vi "FOCUS_V42_H37.vi"(9 "X-pixels":sgl=256.0, 11 "Run":bool) -> (0 "Retrace pixels":sgl, 10 "Pixel Clock (Hz)":sgl)   [LabVIEW 2010] (continued)
                  n1368 = property on="index (row)1" class="Slide (strict)"("Scale.Range:Minimum"=w941, "Scale.Range:Maximum"=w942) -> ()  [unwired: 2 in, 2 out]
                  n1369 = Add(x=w957, y=w958) -> (x+y=w956:dbl)
                  n1370 = property on="Histogram2" class="XYGraph (strict)"("X Scale.Range:Minimum"=w957, "X Scale.Range:Maximum"=w956) -> ()  [unwired: 2 in, 2 out]
                  n1371 = property on="Histogram1" class="XYGraph (strict)"("X Scale.Range:Minimum"=w957, "X Scale.Range:Maximum"=w956) -> ()  [unwired: 2 in, 2 out]
                  n1372 = Initialize Array(u32 0 ("element"), w892) -> (w950:u32[])
                  n1373 = Array Subset(array=w888, index (row)=w903, length (row)=w902) -> (w948:u8[][])  [unwired: 2 in]
                  n1374 = Initialize Array(u32 0 ("element"), w892) -> (w954:u32[])
                  n1375 = Array Subset(array=w887, index (row)=w901, length (row)=w900) -> (w952:u8[][])  [unwired: 2 in]
                  n1376 = property on="index (row)2" class="Slide (strict)"("Scale.Range:Minimum"=w941, "Scale.Range:Maximum"=w940) -> ()  [unwired: 2 in, 2 out]
                  n1377 = local read "Background1"() -> (w914:bool)
                  n1378 = for {
                    tunnel: w948 -> [w1025] mode=indexing
                    shift-right: [w1024] -> w949
                    shift-left: w950 -> [w1026]
                    n1379 = Add(x=w1026, y=w1025) -> (x+y=w1024:u32[])
                  }
                  n1380 = local read "Index1"() -> (w928:dbl)
                  n1381 = local read "Length1"() -> (w929:dbl)
                  n1382 = for {
                    tunnel: w952 -> [w1022] mode=indexing
                    shift-right: [w1021] -> w953
                    shift-left: w954 -> [w1023]
                    n1383 = Add(x=w1023, y=w1022) -> (x+y=w1021:u32[])
                  }
                  n1384 = local read "X-pixels"() -> (w890:sgl)
                  n1385 = local read "Pixel Clock (Hz)"() -> (w946:sgl)
                  n1386 = Divide(x=w949, y=w902) -> (x/y=w891:dbl[])
                  n1387 = Array Subset(array=w891, index=w928, length=w929) -> (w925:dbl[])
                  n1388 = Divide(x=w953, y=w900) -> (x/y=w931:dbl[])
                  n1389 = Array Subset(array=w888, index (row)=w957, length (row)=w958, index (col)=w904, length (col)=w889) -> (w960:u8[][])
                  n1390 = Array Subset(array=w887, index (row)=w957, length (row)=w958, index (col)=w904, length (col)=w889) -> (w959:u8[][])
                  n1391 = case shown="True" w914 {
                    tunnel: w891 -> [_ w968]
                    frame False {
                    }
                    frame True {
                      n1392 = Array Size(array=w968) -> (size(s)=w969:i32)
                      n1393 = Add Array Elements(numeric array=w968) -> (sum=w970:dbl)
                      n1394 = Divide(x=w970, y=w969) -> (x/y=w967:dbl)
                      n1395 = local write "Background1 2"(w967) -> ()
                    }
                  }
                  n1396 = Array Size(array=w925) -> (size(s)=w927:i32)
                  n1397 = Add Array Elements(numeric array=w925) -> (sum=w926:dbl)
                  n1398 = Divide(x=w890, y=w946) -> (x/y=w945:sgl)
                  n1399 = local write "Image 1"(w960) -> ()
                  n1400 = Divide(x=w926, y=w927) -> (x/y=w913:dbl)
                  n1401 = local write "Image 2"(w959) -> ()
                  n1402 = local write "F01 2"(w913) -> ()
                  n1403 = Multiply(x=1000.0, y=w945) -> (x*y=w895:dbl)
                  n1404 = Multiply(x=w892, y=w895) -> (x*y=w937:dbl)
                  n1405 = case shown="True" w915 {
                    tunnel: w937 -> [_ w1020]
                    frame False {
                    }
                    frame True {
                      n1406 = property on="Profile1" class="XYGraph (strict)"("X Scale.Range:Minimum"=0.0, "X Scale.Range:Maximum"=w1020, "Y Scale.Range:Minimum"=0.0, "Y Scale.Range:Maximum"=255.0) -> ()  [unwired: 2 in, 2 out]
                    }
                  }
                  n1407 = case shown="True" w916 {
                    tunnel: w937 -> [_ w997]
                    frame False {
                    }
                    frame True {
                      n1408 = property on="Profile2" class="XYGraph (strict)"("X Scale.Range:Minimum"=0.0, "X Scale.Range:Maximum"=w997, "Y Scale.Range:Minimum"=0.0, "Y Scale.Range:Maximum"=255.0) -> ()  [unwired: 2 in, 2 out]
                    }
                  }
                  n1409 = local read "F0 1"() -> (w908:bool)
                  n1410 = Multiply(x=w895, y=w943) -> (x*y=w897:dbl[])
                  n1411 = Multiply(x=w895, y=w943) -> (x*y=w955:dbl[])
                  n1412 = local read "F0 2"() -> (w909:bool)
                  n1413 = local read "Background2"() -> (w911:bool)
                  n1414 = case shown="True" w909 {
                    tunnel: w931 -> [w1001 w1015]
                    tunnel: [w1001 w1007] -> w939
                    tunnel: w905 -> [w1000 _]
                    tunnel: [w998 i8 -1 ("Active Cursor")] -> w938
                    frame False {
                      n1415 = Less Than 0?(x=w1000) -> (x < 0?=w999:bool)
                      n1416 = case shown="False" w999 {
                        selector: w999 -> [w1003 w1005]
                        tunnel: [i8 1 ("Active Cursor") i8 1 ("Active Cursor")] -> w998
                        frame False {
                          n1417 = local write "Reset2"(w1003) -> ()
                        }
                        frame True {
                          n1418 = local write "Reset2"(w1005) -> ()
                        }
                      }
                    }
                    frame True {
                      n1419 = local read "Background2 2"() -> (w1013:sgl)
                      n1420 = local read "F02 2"() -> (w1010:sgl)
                      n1421 = Subtract(x=w1015, y=w1010) -> (x-y=w1014:dbl[])
                      n1422 = Subtract(x=w1010, y=w1013) -> (x-y=w1016:sgl)
                      n1423 = Divide(x=w1014, y=w1016) -> (x/y=w1008:dbl[])
                      n1424 = property on="Profile2" class="XYGraph (strict)"("Y Scale.Range:Minimum"=-100.0, "Y Scale.Range:Maximum"=100.0) -> ()  [unwired: 2 in, 2 out]
                      n1425 = Multiply(x=w1008, y=100.0 ("Y Scale.Range:Maximum")) -> (x*y=w1007:dbl[])
                    }
                  }
                  n1426 = case shown="True" w908 {
                    tunnel: w891 -> [w974 w988]
                    tunnel: [w974 w980] -> w896
                    tunnel: w906 -> [w973 _]
                    tunnel: [w971 i8 -1 ("Active Cursor")] -> w930
                    frame False {
                      n1427 = Less Than 0?(x=w973) -> (x < 0?=w972:bool)
                      n1428 = case shown="True" w972 {
                        selector: w972 -> [w976 w978]
                        tunnel: [i8 1 ("Active Cursor") i8 1 ("Active Cursor")] -> w971
                        frame False {
                          n1429 = local write "Reset1"(w976) -> ()
                        }
                        frame True {
                          n1430 = local write "Reset1"(w978) -> ()
                        }
                      }
                    }
                    frame True {
                      n1431 = local read "Background1 2"() -> (w986:sgl)
                      n1432 = local read "F01 2"() -> (w983:sgl)
                      n1433 = Subtract(x=w988, y=w983) -> (x-y=w987:dbl[])
                      n1434 = Subtract(x=w983, y=w986) -> (x-y=w989:sgl)
                      n1435 = Divide(x=w987, y=w989) -> (x/y=w981:dbl[])
                      n1436 = property on="Profile1" class="XYGraph (strict)"("Y Scale.Range:Minimum"=-100.0, "Y Scale.Range:Maximum"=100.0) -> ()  [unwired: 2 in, 2 out]
                      n1437 = Multiply(x=w981, y=100.0 ("Y Scale.Range:Maximum")) -> (x*y=w980:dbl[])
                    }
                  }
                  n1438 = property on="Profile2" class="XYGraph (strict)"() -> ("X Scale.Range:Minimum"=w920:dbl, "X Scale.Range:Maximum"=w919:dbl)  [unwired: 2 in, 2 out]
                  n1439 = local read "Index2"() -> (w933:dbl)
                  n1440 = local read "Length2"() -> (w932:dbl)
                  n1441 = property on="Profile1" class="XYGraph (strict)"() -> ("X Scale.Range:Minimum"=w921:dbl, "X Scale.Range:Maximum"=w922:dbl)  [unwired: 2 in, 2 out]
                  n1442 = case shown="True" w911 {
                    tunnel: w931 -> [_ w991]
                    frame False {
                    }
                    frame True {
                      n1443 = Array Size(array=w991) -> (size(s)=w992:i32)
                      n1444 = Add Array Elements(numeric array=w991) -> (sum=w993:dbl)
                      n1445 = Divide(x=w993, y=w992) -> (x/y=w990:dbl)
                      n1446 = local write "Background2 2"(w990) -> ()
                    }
                  }
                  n1447 = Array Subset(array=w931, index=w933, length=w932) -> (w936:dbl[])
                  n1448 = local read "F02"() -> (w907:bool)
                  n1449 = local read "F01"() -> (w912:bool)
                  n1450 = Divide(x=w920, y=w895) -> (x/y=w918:dbl)
                  n1451 = Divide(x=w919, y=w895) -> (x/y=w917:dbl)
                  n1452 = Divide(x=w921, y=w895) -> (x/y=w923:dbl)
                  n1453 = Divide(x=w922, y=w895) -> (x/y=w924:dbl)
                  n1454 = Array Size(array=w936) -> (size(s)=w934:i32)
                  n1455 = Add Array Elements(numeric array=w936) -> (sum=w935:dbl)
                  n1456 = case shown="True" w907 {
                    tunnel: w918 -> [_ w962]
                    tunnel: w917 -> [_ w963]
                    frame False {
                    }
                    frame True {
                      n1457 = local write "Index2"(w962) -> ()
                      n1458 = Subtract(x=w963, y=w962) -> (x-y=w961:dbl)
                      n1459 = local write "Length2"(w961) -> ()
                    }
                  }
                  n1460 = case shown="True" w912 {
                    tunnel: w923 -> [_ w965]
                    tunnel: w924 -> [_ w966]
                    frame False {
                    }
                    frame True {
                      n1461 = Subtract(x=w966, y=w965) -> (x-y=w964:dbl)
                      n1462 = local write "Index1"(w965) -> ()
                      n1463 = local write "Length1"(w964) -> ()
                    }
                  }
                  n1464 = Divide(x=w935, y=w934) -> (x/y=w910:dbl)
                  n1465 = local write "F02 2"(w910) -> ()
                  n1466 = Bundle(w955, w939) -> (w899:cluster{dbl[], dbl[]})  [unwired: 1 in]
                  n1467 = local write "Profile2"(w899) -> ()
                  n1468 = Bundle(w897, w896) -> (w898:cluster{dbl[], dbl[]})  [unwired: 1 in]
                  n1469 = local write "Profile1"(w898) -> ()
                }
                frame True {
                  n1470 = local read "Y-Scale"() -> (w1029:bool)
                  n1471 = case shown="False" w1029 {
                    tunnel: w1028 -> [w1031 _]
                    tunnel: w1027 -> [w1030 _]
                    frame False {
                      n1472 = local read "Y-lines"() -> (w1033:sgl)
                      n1473 = local read "Number of frames"() -> (w1034:sgl)
                      n1474 = local read "X-pixels"() -> (w1036:sgl)
                      n1475 = Multiply(x=w1034, y=w1033) -> (x*y=w1032:sgl)
                      n1476 = Subtract(x=w1032, y=w1036) -> (x-y=w1035:sgl)
                      n1477 = while {
                        shift-right: [w1045] -> _
                        shift-left: i16 0 ("y") -> [w1046]
                        tunnel: w1035 -> [w1044]
                        tunnel: w1031 -> [w1039]
                        tunnel: w1030 -> [w1038]
                        stop <- w1042 stop-if-true
                        n1478 = call "ResetToZeroFOCUS.vi"("UpperLimit"=w1044, "Running Index"=w1046) -> ("New Index"=w1040:i32)
                        n1479 = local read "Play Movie"() -> (w1043:bool)
                        n1480 = local write "ImageSlide"(w1040) -> ()
                        n1481 = local read "X-pixels"() -> (w1049:sgl)
                        n1482 = Not(x=w1043) -> (.not. x?=w1042:bool)
                        n1483 = Increment(x=w1040) -> (x+1=w1045:i32)
                        n1484 = local read "Velocity"() -> (w1041:dbl)
                        n1485 = Array Subset(array=w1039, index (col)=w1040, length (col)=w1049) -> (w1048:u8[][])  [unwired: 2 in]
                        n1486 = Array Subset(array=w1038, index (col)=w1040, length (col)=w1049) -> (w1047:u8[][])  [unwired: 2 in]
                        n1487 = Wait Until Next ms Multiple(millisecond multiple=w1041) -> ()  [unwired: 1 out]
                        n1488 = local write "Image 1"(w1048) -> ()
                        n1489 = local write "Image 2"(w1047) -> ()
                      }
                    }
                    frame True {
                    }
                  }
                }
              }
            }
            frame 3 {
              n1490 = case shown="False" w1056 {
                tunnel: w1055 -> [_ _]
                tunnel: w1061 -> [w1120 _]
                tunnel: [w1114 _] -> w1058
                tunnel: [w1106 _] -> w1057
                tunnel: w1060 -> [w1075 _]
                tunnel: w1059 -> [w1074 _]
                tunnel: w1054 -> [w1066 _]
                tunnel: w1053 -> [w1065 w1206]
                tunnel: w1052 -> [w1064 w1205]
                tunnel: w1051 -> [w1063 _]
                tunnel: w1050 -> [w1062 _]
                frame False {
                  w1067 = 0 ("index")
                  w1135 = 0.0
                  w1118 = 0.0 ("Scale.Range:Minimum")
                  n1491 = local read "Reset1"() -> (w1090:bool)
                  n1492 = local read "Reset2"() -> (w1091:bool)
                  n1493 = local read "Y-lines FreeLine"() -> (w1116:sgl)
                  n1494 = local read "X-pixels FreeLine"() -> (w1136:sgl)
                  n1495 = Add(x=w1135, y=w1136) -> (x+y=w1134:dbl)
                  n1496 = property on="Histogram2" class="XYGraph (strict)"("X Scale.Range:Minimum"=w1135, "X Scale.Range:Maximum"=w1134) -> ()  [unwired: 2 in, 2 out]
                  n1497 = property on="Histogram1" class="XYGraph (strict)"("X Scale.Range:Minimum"=w1135, "X Scale.Range:Maximum"=w1134) -> ()  [unwired: 2 in, 2 out]
                  n1498 = Initialize Array(u32 0 ("element"), w1116) -> (w1128:u32[])
                  n1499 = Array Subset(array=w1065, index (row)="index (row)1", length (row)="Average1") -> (w1126:u8[][])  [unwired: 2 in]
                  n1500 = Initialize Array(u32 0 ("element"), w1116) -> (w1132:u32[])
                  n1501 = Array Subset(array=w1064, index (row)="index (row)2", length (row)="Average2") -> (w1130:u8[][])  [unwired: 2 in]
                  n1502 = local read "Background1"() -> (w1089:bool)
                  n1503 = for {
                    tunnel: w1126 -> [w1203] mode=indexing
                    shift-right: [w1202] -> w1127
                    shift-left: w1128 -> [w1204]
                    n1504 = Add(x=w1204, y=w1203) -> (x+y=w1202:u32[])
                  }
                  n1505 = local read "Index1"() -> (w1104:dbl)
                  n1506 = local read "Length1"() -> (w1105:dbl)
                  n1507 = for {
                    tunnel: w1130 -> [w1200] mode=indexing
                    shift-right: [w1199] -> w1131
                    shift-left: w1132 -> [w1201]
                    n1508 = Add(x=w1201, y=w1200) -> (x+y=w1199:u32[])
                  }
                  n1509 = local read "X-pixels FreeLine"() -> (w1068:sgl)
                  n1510 = Subtract(x=w1068, y="Average2") -> (x-y=w1117:sgl)
                  n1511 = Subtract(x=w1068, y="Average1") -> (x-y=w1119:sgl)
                  n1512 = property on="index (row)1" class="Slide (strict)"("Scale.Range:Minimum"=w1118, "Scale.Range:Maximum"=w1119) -> ()  [unwired: 2 in, 2 out]
                  n1513 = property on="index (row)2" class="Slide (strict)"("Scale.Range:Minimum"=w1118, "Scale.Range:Maximum"=w1117) -> ()  [unwired: 2 in, 2 out]
                  n1514 = local read "Pixel Clock (Hz) FreeLine"() -> (w1124:sgl)
                  n1515 = Divide(x=w1127, y="Average1") -> (x/y=w1073:dbl[])
                  n1516 = Array Subset(array=w1073, index=w1104, length=w1105) -> (w1101:dbl[])
                  n1517 = Divide(x=w1131, y="Average2") -> (x/y=w1107:dbl[])
                  n1518 = Array Subset(array=w1065, index (row)=w1135, length (row)=w1136, index (col)=w1066, length (col)=w1068) -> (w1138:u8[][])
                  n1519 = Array Subset(array=w1064, index (row)=w1135, length (row)=w1136, index (col)=w1066, length (col)=w1068) -> (w1137:u8[][])
                  n1520 = case shown="True" w1089 {
                    tunnel: w1073 -> [_ w1146]
                    frame False {
                    }
                    frame True {
                      n1521 = Array Size(array=w1146) -> (size(s)=w1147:i32)
                      n1522 = Add Array Elements(numeric array=w1146) -> (sum=w1148:dbl)
                      n1523 = Divide(x=w1148, y=w1147) -> (x/y=w1145:dbl)
                      n1524 = local write "Background1 2"(w1145) -> ()
                    }
                  }
                  n1525 = Array Size(array=w1101) -> (size(s)=w1103:i32)
                  n1526 = Add Array Elements(numeric array=w1101) -> (sum=w1102:dbl)
                  n1527 = Divide(x=w1068, y=w1124) -> (x/y=w1123:sgl)
                  n1528 = local write "Image 3"(w1138) -> ()
                  n1529 = Divide(x=w1102, y=w1103) -> (x/y=w1088:dbl)
                  n1530 = local write "Image 4"(w1137) -> ()
                  n1531 = local write "F01 2"(w1088) -> ()
                  n1532 = Multiply(x=1000.0, y=w1123) -> (x*y=w1092:dbl)
                  n1533 = Multiply(x=w1116, y=w1092) -> (x*y=w1113:dbl)
                  n1534 = case shown="True" w1090 {
                    tunnel: w1113 -> [_ w1198]
                    frame False {
                    }
                    frame True {
                      n1535 = property on="Profile1" class="XYGraph (strict)"("X Scale.Range:Minimum"=0.0, "X Scale.Range:Maximum"=w1198, "Y Scale.Range:Minimum"=0.0, "Y Scale.Range:Maximum"=255.0) -> ()  [unwired: 2 in, 2 out]
                    }
                  }
                  n1536 = case shown="True" w1091 {
                    tunnel: w1113 -> [_ w1175]
                    frame False {
                    }
                    frame True {
                      n1537 = property on="Profile2" class="XYGraph (strict)"("X Scale.Range:Minimum"=0.0, "X Scale.Range:Maximum"=w1175, "Y Scale.Range:Minimum"=0.0, "Y Scale.Range:Maximum"=255.0) -> ()  [unwired: 2 in, 2 out]
                    }
                  }
                  n1538 = local read "Y-lines"() -> (w1069:sgl)
                  n1539 = local read "F0 1"() -> (w1083:bool)
                  n1540 = Multiply(x=w1092, y=w1120) -> (x*y=w1121:dbl[])
                  n1541 = Multiply(x=w1092, y=w1120) -> (x*y=w1133:dbl[])
                  n1542 = local read "F0 2"() -> (w1084:bool)
                  n1543 = local read "Background2"() -> (w1086:bool)
                  n1544 = case shown="True" w1084 {
                    tunnel: w1107 -> [w1179 w1193]
                    tunnel: [w1179 w1185] -> w1115
                    tunnel: w1074 -> [w1178 _]
                    tunnel: [w1176 i8 -1 ("Active Cursor")] -> w1114
                    frame False {
                      n1545 = Less Than 0?(x=w1178) -> (x < 0?=w1177:bool)
                      n1546 = case shown="True" w1177 {
                        selector: w1177 -> [w1181 w1183]
                        tunnel: [i8 1 ("Active Cursor") i8 1 ("Active Cursor")] -> w1176
                        frame False {
                          n1547 = local write "Reset2"(w1181) -> ()
                        }
                        frame True {
                          n1548 = local write "Reset2"(w1183) -> ()
                        }
                      }
                    }
                    frame True {
                      n1549 = local read "Background2 2"() -> (w1191:sgl)
                      n1550 = local read "F02 2"() -> (w1188:sgl)
                      n1551 = Subtract(x=w1193, y=w1188) -> (x-y=w1192:dbl[])
                      n1552 = Subtract(x=w1188, y=w1191) -> (x-y=w1194:sgl)
                      n1553 = Divide(x=w1192, y=w1194) -> (x/y=w1186:dbl[])
                      n1554 = property on="Profile2" class="XYGraph (strict)"("Y Scale.Range:Minimum"=-100.0, "Y Scale.Range:Maximum"=100.0) -> ()  [unwired: 2 in, 2 out]
                      n1555 = Multiply(x=w1186, y=100.0 ("Y Scale.Range:Maximum")) -> (x*y=w1185:dbl[])
                    }
                  }
                  n1556 = case shown="True" w1083 {
                    tunnel: w1073 -> [w1152 w1166]
                    tunnel: [w1152 w1158] -> w1072
                    tunnel: w1075 -> [w1151 _]
                    tunnel: [w1149 i8 -1 ("Active Cursor")] -> w1106
                    frame False {
                      n1557 = Less Than 0?(x=w1151) -> (x < 0?=w1150:bool)
                      n1558 = case shown="False" w1150 {
                        selector: w1150 -> [w1154 w1156]
                        tunnel: [i8 1 ("Active Cursor") i8 1 ("Active Cursor")] -> w1149
                        frame False {
                          n1559 = local write "Reset1"(w1154) -> ()
                        }
                        frame True {
                          n1560 = local write "Reset1"(w1156) -> ()
                        }
                      }
                    }
                    frame True {
                      n1561 = local read "Background1 2"() -> (w1164:sgl)
                      n1562 = local read "F01 2"() -> (w1161:sgl)
                      n1563 = Subtract(x=w1166, y=w1161) -> (x-y=w1165:dbl[])
                      n1564 = Subtract(x=w1161, y=w1164) -> (x-y=w1167:sgl)
                      n1565 = Divide(x=w1165, y=w1167) -> (x/y=w1159:dbl[])
                      n1566 = property on="Profile1" class="XYGraph (strict)"("Y Scale.Range:Minimum"=-100.0, "Y Scale.Range:Maximum"=100.0) -> ()  [unwired: 2 in, 2 out]
                      n1567 = Multiply(x=w1159, y=100.0 ("Y Scale.Range:Maximum")) -> (x*y=w1158:dbl[])
                    }
                  }
                  n1568 = property on="Profile2" class="XYGraph (strict)"() -> ("X Scale.Range:Minimum"=w1096:dbl, "X Scale.Range:Maximum"=w1095:dbl)  [unwired: 2 in, 2 out]
                  n1569 = Array Subset(array=w1063, index (col)=w1067, length (col)=w1069) -> (w1071:u8[][])  [unwired: 2 in]
                  n1570 = local read "Index2"() -> (w1109:dbl)
                  n1571 = local read "Length2"() -> (w1108:dbl)
                  n1572 = property on="Profile1" class="XYGraph (strict)"() -> ("X Scale.Range:Minimum"=w1097:dbl, "X Scale.Range:Maximum"=w1098:dbl)  [unwired: 2 in, 2 out]
                  n1573 = local write "Image 1"(w1071) -> ()
                  n1574 = case shown="True" w1086 {
                    tunnel: w1107 -> [_ w1169]
                    frame False {
                    }
                    frame True {
                      n1575 = Array Size(array=w1169) -> (size(s)=w1170:i32)
                      n1576 = Add Array Elements(numeric array=w1169) -> (sum=w1171:dbl)
                      n1577 = Divide(x=w1171, y=w1170) -> (x/y=w1168:dbl)
                      n1578 = local write "Background2 2"(w1168) -> ()
                    }
                  }
                  n1579 = Array Subset(array=w1107, index=w1109, length=w1108) -> (w1112:dbl[])
                  n1580 = local read "F02"() -> (w1082:bool)
                  n1581 = local read "F01"() -> (w1087:bool)
                  n1582 = Divide(x=w1096, y=w1092) -> (x/y=w1094:dbl)
                  n1583 = Divide(x=w1095, y=w1092) -> (x/y=w1093:dbl)
                  n1584 = Divide(x=w1097, y=w1092) -> (x/y=w1099:dbl)
                  n1585 = Divide(x=w1098, y=w1092) -> (x/y=w1100:dbl)
                  n1586 = Array Size(array=w1112) -> (size(s)=w1110:i32)
                  n1587 = Add Array Elements(numeric array=w1112) -> (sum=w1111:dbl)
                  n1588 = case shown="True" w1082 {
                    tunnel: w1094 -> [_ w1140]
                    tunnel: w1093 -> [_ w1141]
                    frame False {
                    }
                    frame True {
                      n1589 = local write "Index2"(w1140) -> ()
                      n1590 = Subtract(x=w1141, y=w1140) -> (x-y=w1139:dbl)
                      n1591 = local write "Length2"(w1139) -> ()
                    }
                  }
                  n1592 = case shown="True" w1087 {
                    tunnel: w1099 -> [_ w1143]
                    tunnel: w1100 -> [_ w1144]
                    frame False {
                    }
                    frame True {
                      n1593 = Subtract(x=w1144, y=w1143) -> (x-y=w1142:dbl)
                      n1594 = local write "Index1"(w1143) -> ()
                      n1595 = local write "Length1"(w1142) -> ()
                    }
                  }
                  n1596 = Divide(x=w1111, y=w1110) -> (x/y=w1085:dbl)
                  n1597 = Array Subset(array=w1062, index (col)=w1067, length (col)=w1069) -> (w1070:u8[][])  [unwired: 2 in]
                  n1598 = local write "F02 2"(w1085) -> ()
                  n1599 = local write "Image 2"(w1070) -> ()
                  n1600 = Bundle(w1133, w1115) -> (→"Profile2":cluster{dbl[], dbl[]})  [unwired: 1 in]
                  n1601 = Bundle(w1121, w1072) -> (→"Profile1":cluster{dbl[], dbl[]})  [unwired: 1 in]
                }
                frame True {
                  n1602 = local read "X-pixels FreeLine"() -> (w1209:sgl)
                  n1603 = local read "Y-lines FreeLine"() -> (w1207:sgl)
                  n1604 = Subtract(x=w1207, y=w1209) -> (x-y=w1208:sgl)
                  n1605 = while {
                    shift-right: [w1219] -> _
                    shift-left: i16 0 ("y") -> [w1220]
                    tunnel: w1208 -> [w1218]
                    tunnel: w1207 -> [w1214]
                    tunnel: w1206 -> [w1212]
                    tunnel: w1205 -> [w1211]
                    stop <- w1216 stop-if-true
                    n1606 = call "ResetToZeroFOCUS.vi"("UpperLimit"=w1218, "Running Index"=w1220) -> ("New Index"=w1213:i32)
                    n1607 = Multiply(x=w1213, y=w1214) -> ()  [unwired: 1 out]
                    n1608 = local read "Play Movie"() -> (w1217:bool)
                    n1609 = local write "ImageSlide"(w1213) -> ()
                    n1610 = local read "X-pixels FreeLine"() -> (w1223:sgl)
                    n1611 = Not(x=w1217) -> (.not. x?=w1216:bool)
                    n1612 = Increment(x=w1213) -> (x+1=w1219:i32)
                    n1613 = local read "Velocity"() -> (w1215:dbl)
                    n1614 = Array Subset(array=w1212, index (col)=w1213, length (col)=w1223) -> (w1222:u8[][])  [unwired: 2 in]
                    n1615 = Array Subset(array=w1211, index (col)=w1213, length (col)=w1223) -> (w1221:u8[][])  [unwired: 2 in]
                    n1616 = Wait Until Next ms Multiple(millisecond multiple=w1215) -> ()  [unwired: 1 out]
                    n1617 = local write "Image 3"(w1222) -> ()
                    n1618 = local write "Image 4"(w1221) -> ()
                  }
                }
              }
            }
            frame 4 {
              n1619 = case shown="False" w1234 {
                tunnel: w1235 -> [w1240 _]
                tunnel: w1233 -> [w1315 _]
                tunnel: w1232 -> [w1295 _]
                tunnel: w1231 -> [w1281 _]
                tunnel: [w1280 _] -> w1230
                tunnel: w1229 -> [w1269 _]
                tunnel: [w1268 _] -> w1228
                tunnel: w1227 -> [w1239 w1389]
                tunnel: w1226 -> [w1238 w1388]
                tunnel: w1225 -> [w1237 _]
                tunnel: w1224 -> [w1236 _]
                frame False {
                  w1292 = 0.0 ("Scale.Range:Minimum")
                  n1620 = local read "index (row)2"() -> (w1290:i32)
                  n1621 = local read "XScale"() -> (w1314:bool)
                  n1622 = local read "index (row)1"() -> (w1288:i32)
                  n1623 = Round To Nearest(number=w1315) -> (nearest integer value=w1313:u32)
                  n1624 = local read "Y-lines FreeLine"() -> (w1284:sgl)
                  n1625 = case shown="False" w1314 {
                    tunnel: [w1385 w1387] -> w1312
                    tunnel: w1313 -> [w1384 _]
                    tunnel: [w1384 0.0] -> w1311
                    frame False {
                      n1626 = local read "Y-lines FreeLine"() -> (w1385:sgl)
                    }
                    frame True {
                      n1627 = local read "X-pixels FreeLine"() -> (w1387:sgl)
                    }
                  }
                  n1628 = local read "Average2"() -> (w1287:i32)
                  n1629 = local read "Average1"() -> (w1286:i32)
                  n1630 = Add(x=w1311, y=w1312) -> (x+y=w1310:dbl)
                  n1631 = property on="Histogram2" class="XYGraph (strict)"("X Scale.Range:Minimum"=w1311, "X Scale.Range:Maximum"=w1310) -> ()  [unwired: 2 in, 2 out]
                  n1632 = property on="Histogram1" class="XYGraph (strict)"("X Scale.Range:Minimum"=w1311, "X Scale.Range:Maximum"=w1310) -> ()  [unwired: 2 in, 2 out]
                  n1633 = Initialize Array(u32 0 ("element"), w1284) -> (w1304:u32[])
                  n1634 = Array Subset(array=w1239, index (row)=w1288, length (row)=w1286) -> (w1302:u8[][])  [unwired: 2 in]
                  n1635 = Initialize Array(u32 0 ("element"), w1284) -> (w1308:u32[])
                  n1636 = Array Subset(array=w1238, index (row)=w1290, length (row)=w1287) -> (w1306:u8[][])  [unwired: 2 in]
                  n1637 = for {
                    tunnel: w1302 -> [w1382] mode=indexing
                    shift-right: [w1381] -> w1303
                    shift-left: w1304 -> [w1383]
                    n1638 = Add(x=w1383, y=w1382) -> (x+y=w1381:u32[])
                  }
                  n1639 = local read "Index1"() -> (w1264:dbl)
                  n1640 = local read "Length1"() -> (w1265:dbl)
                  n1641 = for {
                    tunnel: w1306 -> [w1379] mode=indexing
                    shift-right: [w1378] -> w1307
                    shift-left: w1308 -> [w1380]
                    n1642 = Add(x=w1380, y=w1379) -> (x+y=w1378:u32[])
                  }
                  n1643 = local read "X-pixels FreeLine"() -> (w1291:sgl)
                  n1644 = Subtract(x=w1291, y=w1287) -> (x-y=w1289:sgl)
                  n1645 = Subtract(x=w1291, y=w1286) -> (x-y=w1293:sgl)
                  n1646 = property on="index (row)1" class="Slide (strict)"("Scale.Range:Minimum"=w1292, "Scale.Range:Maximum"=w1293) -> ()  [unwired: 2 in, 2 out]
                  n1647 = property on="index (row)2" class="Slide (strict)"("Scale.Range:Minimum"=w1292, "Scale.Range:Maximum"=w1289) -> ()  [unwired: 2 in, 2 out]
                  n1648 = local read "Pixel Clock (Hz) FreeLine"() -> (w1300:sgl)
                  n1649 = Divide(x=w1303, y=w1286) -> (x/y=w1248:dbl[])
                  n1650 = Array Subset(array=w1248, index=w1264, length=w1265) -> (w1260:dbl[])
                  n1651 = Divide(x=w1307, y=w1287) -> (x/y=w1270:dbl[])
                  n1652 = Array Subset(array=w1239, index (row)=w1311, length (row)=w1312) -> (w1317:u8[][])  [unwired: 2 in]
                  n1653 = Array Subset(array=w1238, index (row)=w1311, length (row)=w1312) -> (w1316:u8[][])  [unwired: 2 in]
                  n1654 = local read "Y-lines"() -> (w1246:sgl)
                  n1655 = case shown="True" "Background1" {
                    tunnel: w1248 -> [_ w1325]
                    frame False {
                    }
                    frame True {
                      n1656 = Array Size(array=w1325) -> (size(s)=w1326:i32)
                      n1657 = Add Array Elements(numeric array=w1325) -> (sum=w1327:dbl)
                      n1658 = Divide(x=w1327, y=w1326) -> (x/y=→"Background1 2":dbl)
                    }
                  }
                  n1659 = Array Size(array=w1260) -> (size(s)=w1263:i32)
                  n1660 = Add Array Elements(numeric array=w1260) -> (sum=w1262:dbl)
                  n1661 = Round To Nearest(number=w1240) -> (nearest integer value=w1245:u32)
                  n1662 = Divide(x=w1291, y=w1300) -> (x/y=w1299:sgl)
                  n1663 = local write "Image 3"(w1317) -> ()
                  n1664 = Divide(x=w1262, y=w1263) -> (x/y=→"F01 2":dbl)
                  n1665 = local write "Image 4"(w1316) -> ()
                  n1666 = Multiply(x=w1246, y=w1245) -> (x*y=w1241:sgl)
                  n1667 = local read "Y-lines"() -> (w1242:sgl)
                  n1668 = Multiply(x=1000.0, y=w1299) -> (x*y=w1249:dbl)
                  n1669 = Multiply(x=w1284, y=w1249) -> (x*y=w1279:dbl)
                  n1670 = case shown="True" "Reset1" {
                    tunnel: w1279 -> [_ w1377]
                    frame False {
                    }
                    frame True {
                      n1671 = property on="Profile1" class="XYGraph (strict)"("X Scale.Range:Minimum"=0.0, "X Scale.Range:Maximum"=w1377, "Y Scale.Range:Minimum"=0.0, "Y Scale.Range:Maximum"=255.0) -> ()  [unwired: 2 in, 2 out]
                    }
                  }
                  n1672 = case shown="True" "Reset2" {
                    tunnel: w1279 -> [_ w1354]
                    frame False {
                    }
                    frame True {
                      n1673 = property on="Profile2" class="XYGraph (strict)"("X Scale.Range:Minimum"=0.0, "X Scale.Range:Maximum"=w1354, "Y Scale.Range:Minimum"=0.0, "Y Scale.Range:Maximum"=255.0) -> ()  [unwired: 2 in, 2 out]
                    }
                  }
                  n1674 = Multiply(x=w1249, y=w1295) -> (x*y=w1296:dbl[])
                  n1675 = Multiply(x=w1249, y=w1295) -> (x*y=w1309:dbl[])
                  n1676 = Array Subset(array=w1237, index (col)=w1241, length (col)=w1242) -> (w1244:u8[][])  [unwired: 2 in]
                  n1677 = case shown="True" "F0 1" {
                    tunnel: w1248 -> [w1331 w1345]
                    tunnel: [w1331 w1337] -> w1247
                    tunnel: w1269 -> [w1330 _]
                    tunnel: [w1328 i8 -1 ("Active Cursor")] -> w1268
                    frame False {
                      n1678 = Less Than 0?(x=w1330) -> (x < 0?=w1329:bool)
                      n1679 = case shown="True" w1329 {
                        selector: w1329 -> [w1333 w1335]
                        tunnel: [i8 1 ("Active Cursor") i8 1 ("Active Cursor")] -> w1328
                        frame False {
                          n1680 = local write "Reset1"(w1333) -> ()
                        }
                        frame True {
                          n1681 = local write "Reset1"(w1335) -> ()
                        }
                      }
                    }
                    frame True {
                      n1682 = local read "Background1 2"() -> (w1343:sgl)
                      n1683 = local read "F01 2"() -> (w1340:sgl)
                      n1684 = Subtract(x=w1345, y=w1340) -> (x-y=w1344:dbl[])
                      n1685 = Subtract(x=w1340, y=w1343) -> (x-y=w1346:sgl)
                      n1686 = Divide(x=w1344, y=w1346) -> (x/y=w1338:dbl[])
                      n1687 = property on="Profile1" class="XYGraph (strict)"("Y Scale.Range:Minimum"=-100.0, "Y Scale.Range:Maximum"=100.0) -> ()  [unwired: 2 in, 2 out]
                      n1688 = Multiply(x=w1338, y=100.0 ("Y Scale.Range:Maximum")) -> (x*y=w1337:dbl[])
                    }
                  }
                  n1689 = case shown="True" "F0 2" {
                    tunnel: w1270 -> [w1358 w1372]
                    tunnel: [w1358 w1364] -> w1282
                    tunnel: w1281 -> [w1357 _]
                    tunnel: [w1355 i8 -1 ("Active Cursor")] -> w1280
                    frame False {
                      n1690 = Less Than 0?(x=w1357) -> (x < 0?=w1356:bool)
                      n1691 = case shown="False" w1356 {
                        selector: w1356 -> [w1360 w1362]
                        tunnel: [i8 1 ("Active Cursor") i8 1 ("Active Cursor")] -> w1355
                        frame False {
                          n1692 = local write "Reset2"(w1360) -> ()
                        }
                        frame True {
                          n1693 = local write "Reset2"(w1362) -> ()
                        }
                      }
                    }
                    frame True {
                      n1694 = local read "Background2 2"() -> (w1370:sgl)
                      n1695 = local read "F02 2"() -> (w1367:sgl)
                      n1696 = Subtract(x=w1372, y=w1367) -> (x-y=w1371:dbl[])
                      n1697 = Subtract(x=w1367, y=w1370) -> (x-y=w1373:sgl)
                      n1698 = Divide(x=w1371, y=w1373) -> (x/y=w1365:dbl[])
                      n1699 = property on="Profile2" class="XYGraph (strict)"("Y Scale.Range:Minimum"=-100.0, "Y Scale.Range:Maximum"=100.0) -> ()  [unwired: 2 in, 2 out]
                      n1700 = Multiply(x=w1365, y=100.0 ("Y Scale.Range:Maximum")) -> (x*y=w1364:dbl[])
                    }
                  }
                  n1701 = local read "Index2"() -> (w1273:dbl)
                  n1702 = local read "Length2"() -> (w1272:dbl)
                  n1703 = property on="Profile1" class="XYGraph (strict)"() -> ("X Scale.Range:Minimum"=w1255:dbl, "X Scale.Range:Maximum"=w1256:dbl)  [unwired: 2 in, 2 out]
                  n1704 = local write "Image 1"(w1244) -> ()
                  n1705 = property on="Profile2" class="XYGraph (strict)"() -> ("X Scale.Range:Minimum"=w1254:dbl, "X Scale.Range:Maximum"=w1253:dbl)  [unwired: 2 in, 2 out]
                  n1706 = case shown="True" "Background2" {
                    tunnel: w1270 -> [_ w1348]
                    frame False {
                    }
                    frame True {
                      n1707 = Array Size(array=w1348) -> (size(s)=w1349:i32)
                      n1708 = Add Array Elements(numeric array=w1348) -> (sum=w1350:dbl)
                      n1709 = Divide(x=w1350, y=w1349) -> (x/y=→"Background2 2":dbl)
                    }
                  }
                  n1710 = Array Subset(array=w1270, index=w1273, length=w1272) -> (w1277:dbl[])
                  n1711 = Divide(x=w1255, y=w1249) -> (x/y=w1258:dbl)
                  n1712 = Divide(x=w1256, y=w1249) -> (x/y=w1259:dbl)
                  n1713 = Array Size(array=w1277) -> (size(s)=w1274:i32)
                  n1714 = Add Array Elements(numeric array=w1277) -> (sum=w1275:dbl)
                  n1715 = Divide(x=w1254, y=w1249) -> (x/y=w1251:dbl)
                  n1716 = Divide(x=w1253, y=w1249) -> (x/y=w1250:dbl)
                  n1717 = case shown="True" "F01" {
                    tunnel: w1258 -> [_ w1322]
                    tunnel: w1259 -> [_ w1323]
                    frame False {
                    }
                    frame True {
                      n1718 = Subtract(x=w1323, y=w1322) -> (x-y=→"Length1":dbl)
                      "Index1" <- w1322
                    }
                  }
                  n1719 = Divide(x=w1275, y=w1274) -> (x/y=→"F02 2":dbl)
                  n1720 = Array Subset(array=w1236, index (col)=w1241, length (col)=w1242) -> (w1243:u8[][])  [unwired: 2 in]
                  n1721 = case shown="True" "F02" {
                    tunnel: w1251 -> [_ w1319]
                    tunnel: w1250 -> [_ w1320]
                    frame False {
                    }
                    frame True {
                      n1722 = Subtract(x=w1320, y=w1319) -> (x-y=→"Length2":dbl)
                      "Index2" <- w1319
                    }
                  }
                  n1723 = local write "Image 2"(w1243) -> ()
                  n1724 = Bundle(w1309, w1282) -> (w1297:cluster{dbl[], dbl[]})  [unwired: 1 in]
                  n1725 = local write "Profile2"(w1297) -> ()
                  n1726 = Bundle(w1296, w1247) -> (w1294:cluster{dbl[], dbl[]})  [unwired: 1 in]
                  n1727 = local write "Profile1"(w1294) -> ()
                }
                frame True {
                  n1728 = local read "X-pixels FreeLine"() -> (w1392:sgl)
                  n1729 = local read "Y-lines FreeLine"() -> (w1390:sgl)
                  n1730 = Subtract(x=w1390, y=w1392) -> (x-y=w1391:sgl)
                  n1731 = while {
                    shift-right: [w1402] -> _
                    shift-left: i16 0 ("y") -> [w1403]
                    tunnel: w1391 -> [w1401]
                    tunnel: w1390 -> [w1397]
                    tunnel: w1389 -> [w1395]
                    tunnel: w1388 -> [w1394]
                    stop <- w1399 stop-if-true
                    n1732 = call "ResetToZeroFOCUS.vi"("UpperLimit"=w1401, "Running Index"=w1403) -> ("New Index"=w1396:i32)
                    n1733 = Multiply(x=w1396, y=w1397) -> ()  [unwired: 1 out]
                    n1734 = local read "Play Movie"() -> (w1400:bool)
                    n1735 = local write "ImageSlide"(w1396) -> ()
                    n1736 = local read "Y-lines FreeLine"() -> (w1406:sgl)
                    n1737 = Not(x=w1400) -> (.not. x?=w1399:bool)
                    n1738 = Increment(x=w1396) -> (x+1=w1402:i32)
                    n1739 = local read "Velocity"() -> (w1398:dbl)
                    n1740 = Array Subset(array=w1395, index (col)=w1396, length (col)=w1406) -> (w1405:u8[][])  [unwired: 2 in]
                    n1741 = Array Subset(array=w1394, index (col)=w1396, length (col)=w1406) -> (w1404:u8[][])  [unwired: 2 in]
                    n1742 = Wait Until Next ms Multiple(millisecond multiple=w1398) -> ()  [unwired: 1 out]
                    n1743 = local write "Image 3"(w1405) -> ()
                    n1744 = local write "Image 4"(w1404) -> ()
                  }
                }
              }
            }
          }
          n1745 = property on="Image 2" class="IntGraph (strict)"("Y Scale.Range:Maximum"=w500) -> ()  [unwired: 2 in, 2 out]
          n1746 = property on="SlideHorizontal" class="Slide (strict)"("Visible"=w570) -> ()  [unwired: 2 in, 2 out]
          n1747 = case shown="True" w520 {
            tunnel: w531 -> [_ w818]
            tunnel: "ImageSelector" -> [_ w816]
            tunnel: [w815 w816] -> w529
            tunnel: w528 -> [w815 _]
            frame False {
            }
            frame True {
              n1748 = Round Toward +Infinity(x=w818) -> (ceil(x): smallest int >= x=w817:dbl)
              n1749 = local write "ImageSlide"(w817) -> ()
            }
          }
          n1750 = case shown="True" "Zero 2" {
            tunnel: [w813 w814] -> w513
            frame False {
              n1751 = global read "GlobelFSCOPE.vi" "Focus"() -> (w813:dbl)
            }
            frame True {
              w814 = 0.0 ("Focus")
              n1752 = global write "GlobelFSCOPE.vi" "Focus"(w814) -> ()
            }
          }
          "Focus" <- w513
          n1753 = property on="Image 1" class="IntGraph (strict)"("Y Scale.Range:Maximum"=w500) -> ()  [unwired: 2 in, 2 out]
          n1754 = property on="ImageSlide" class="Slide (strict)"("Scale.Range:Minimum"=0.0, "Scale.Range:Maximum"=w531, "Visible"=w535) -> ()  [unwired: 2 in, 2 out]
          n1755 = Wait (ms)(milliseconds to wait=u32 40) -> ()  [unwired: 1 out]
          "Ready?" <- TRUE ("Ready?")
        }
        "Intensity" <- w398
      }
    }
    n1756 = local read "ParametersFScope"() -> (w221:T7)
    n1757 = local read "scans to read"() -> (w222:sgl)
    n1758 = local read "ScaleCluster"() -> (w223:T3)
    n1759 = Bundle("ScaleCluster"=w223, "scans to read"=w222) -> (w220:T20)  [unwired: 1 in]
    n1760 = call "ScaleScanlineFScope.vi"("Parameters"=w221, "ScaleCluster"=w220) -> ("ScanlineScaled"=w215:dbl[][])
    n1761 = case shown="True" w210 {
      tunnel: [w340 w343] -> w211
      frame False {
        n1762 = local read "line scan time (ms)"() -> (w342:sgl)
        n1763 = local read "total y pixels"() -> (w341:sgl)
        n1764 = Multiply(x=w342, y=w341) -> (x*y=w340:sgl)
      }
      frame True {
        n1765 = local read "Pixel Clock (Hz) FScope"() -> (w345:sgl)
        n1766 = local read "scans to read"() -> (w344:sgl)
        n1767 = Divide(x=w344, y=w345) -> (x/y=w343:sgl)
      }
    }
    n1768 = local read "Number of frames"() -> (w213:sgl)
    n1769 = local read "Averaging"() -> (w214:u16)
    n1770 = Compound Arithmetic op=MULTIPLY(w213, w214, w211) -> (w212:sgl)
    n1771 = case shown="True" w296 {
      tunnel: w287 -> [w3060 w3267]
      tunnel: w286 -> [w3061 w3266]
      tunnel: w290 -> [w3059 w3243]
      tunnel: w260 -> [w3058 w3244]
      tunnel: w298 -> [w3055 w3294]
      tunnel: w262 -> [w3056 w3293]
      tunnel: w297 -> [w3057 w3292]
      tunnel: [w3055 w3291] -> w268
      tunnel: [w3056 w3290] -> w267
      tunnel: [w3057 w3289] -> w266
      tunnel: [w3058 w3288] -> w278
      tunnel: [w3059 w3287] -> w280
      tunnel: [w3060 w3286] -> w270
      tunnel: [w3061 w3269] -> w271
      tunnel: [w3053 w3249] -> w294
      tunnel: [w3054 w3250] -> w293
      tunnel: w292 -> [w3054 w3278]
      tunnel: w291 -> [w3053 w3280]
      tunnel: w261 -> [w3052 w3242]
      tunnel: w285 -> [w3051 w3241]
      tunnel: [w3052 w3272] -> w272
      tunnel: [w3051 w3271] -> w224
      tunnel: w277 -> [w3047 w3258]
      tunnel: w276 -> [w3046 w3257]
      tunnel: [w3047 w3256] -> w274
      tunnel: [w3046 w3255] -> w273
      tunnel: w264 -> [w3045 w3254]
      tunnel: [w3045 w3230] -> w199
      tunnel: w221 -> [_ w3238]
      tunnel: w215 -> [_ w3237]
      tunnel: w220 -> [_ w3236]
      tunnel: w219 -> [w3043 w3235]
      tunnel: w218 -> [w3044 w3234]
      tunnel: [w3043 w3233] -> w216
      tunnel: [w3044 w3232] -> w217
      tunnel: w212 -> [_ w3231]
      tunnel: w176 -> [w3040 w3229]
      tunnel: w186 -> [w3039 w3228]
      tunnel: [w3042 w3227] -> w191
      tunnel: [w3041 w3226] -> w190
      tunnel: [w3035 w3225] -> w189
      tunnel: [w3036 w3224] -> w188
      tunnel: w171 -> [w3038 w3223]
      tunnel: w187 -> [w3037 w3222]
      tunnel: w167 -> [_ w3200]
      tunnel: [w3034 w3200] -> w164
      tunnel: w163 -> [w3034 _]
      tunnel: w161 -> [w3033 _]
      frame False {
        n1772 = local write "Ready?"(FALSE ("Ready?")) -> ()
        n1773 = local write "Save?"(FALSE ("Save?")) -> ()
        n1774 = local read "Open?"() -> (w3050:bool)
        n1775 = case shown="False" w3050 {
          tunnel: [w3066 w3142] -> w3042
          tunnel: [w3068 w3141] -> w3041
          tunnel: w3040 -> [w3067 _]
          tunnel: w3039 -> [w3069 _]
          tunnel: [w3070 w3140] -> w3036
          tunnel: [w3071 w3139] -> w3035
          tunnel: w3038 -> [w3071 _]
          tunnel: w3037 -> [w3070 _]
          tunnel: w3033 -> [w3062 _]
          frame False {
            n1776 = local read "Channel selector"() -> (w3063:u8)
            n1777 = Greater Or Equal?(x=w3063, y=u16 3) -> (x >= y?=w3064:bool)
            n1778 = And(x=w3062, y=w3064) -> ()  [unwired: 1 out]
            n1779 = case shown="True" w3062 {
              tunnel: w3067 -> [w3072 _]
              tunnel: w3069 -> [w3073 _]
              tunnel: [w3073 w3078] -> w3068
              tunnel: [w3072 w3077] -> w3066
              tunnel: w3063 -> [_ w3079]
              frame False {
              }
              frame True {
                w3102 = 1  # bytes/DBL
                w3104 = u8 0  # type U8
                n1780 = property on="Property Node" class="VI"() -> ("VI Path"=w3091:path)  [unwired: 2 in, 2 out]
                n1781 = Strip Path(path=w3091) -> (stripped path=w3092:path)  [unwired: 1 out]
                n1782 = Build Path(base path=w3092, name or relative path="Stack.tmp") -> (appended path=w3089:path)
                n1783 = Open/Create/Replace File "Open File"(file path (use dialog)=w3089) -> (refnum out=w3074:refnum<file>, error out=w3075:errorcluster)  [unwired: 5 in, 1 out]
                n1784 = Deny Access(4:w3075, 6:T12."deny write-only" ("deny mode (2)"), 7:w3074) -> (0:w3098:errorcluster, 3:w3099:refnum<file>)
                n1785 = Get File Size "EOF"(file=w3099, error in=w3098) -> (refnum out=w3105:refnum<file>, size (in bytes)=w3076:i64, 0:w3100:errorcluster)
                n1786 = To Long Integer(number=w3076) -> (32bit integer=w3103:i32)
                n1787 = Quotient & Remainder(x=w3103, y=w3102) -> (floor(x/y)=w3101:i32)  [unwired: 1 out]
                n1788 = local read "X-pixels"() -> (w3083:sgl)
                n1789 = Read from Binary File "Read File"(5:w3104, 8:w3100, 10:w3101, 11:w3105) -> (0:w3093:errorcluster, 2:w3096:u8[], 3:w3094:refnum<file>)  [unwired: 2 in, 1 out]
                n1790 = Array Subset(array=w3096, index=768) -> (w3081:u8[])  [unwired: 1 in]
                n1791 = case shown="0, Default" w3079 {
                  tunnel: [w3109 w3112 w3113 w3116 w3120 w3124] -> w3082
                  tunnel: w3081 -> [w3108 w3111 w3115 w3118 w3121 w3123]
                  tunnel: [w3107 w3110 w3114 w3117 w3119 w3122] -> w3080
                  frame 1 {
                    n1792 = Decimate 1D Array(w3108) -> (w3109:u8[], w3107:u8[])
                  }
                  frame 2 {
                    n1793 = Decimate 1D Array(w3111) -> (w3112:u8[], w3110:u8[])
                  }
                  frame 3 {
                    n1794 = Decimate 1D Array(w3115) -> (w3114:u8[], w3113:u8[])  [unwired: 1 out]
                  }
                  frame 4 {
                    n1795 = Decimate 1D Array(w3118) -> (w3116:u8[], w3117:u8[])  [unwired: 1 out]
                  }
                  frame 5 {
                    n1796 = Decimate 1D Array(w3121) -> (w3119:u8[], w3120:u8[])  [unwired: 1 out]
                  }
                  frame 0, Default {
                    n1797 = Decimate 1D Array(w3123) -> (w3124:u8[], w3122:u8[])
                  }
                }
                n1798 = Array Size(array=w3082) -> (size(s)=w3084:i32)
                n1799 = Divide(x=w3084, y=w3083) -> (x/y=w3085:sgl)
                n1800 = Close File(refnum=w3094, error in=w3093) -> (error out=w3095:errorcluster)  [unwired: 1 out]
                n1801 = Round To Nearest(number=w3085) -> (nearest integer value=w3088:sgl)
                n1802 = call <vilib>:"Simple Error Handler.vi"("error in (no error)"=w3095) -> ()  [unwired: 4 in, 5 out]
                n1803 = Reshape Array(w3082, w3088, w3083) -> (w3086:u8[][])
                n1804 = Reshape Array(w3080, w3088, w3083) -> (w3087:u8[][])
                n1805 = Transpose 2D Array(2D array=w3086) -> (transposed array=w3077:u8[][])
                n1806 = Transpose 2D Array(2D array=w3087) -> (transposed array=w3078:u8[][])
              }
            }
          }
          frame True {
            w3174 = u16 1 items=["focus", "frame", "line", "user-defined line", "3D user-defined line"] ("frame/line indicator")
            w3189 = u16 0 items=["user-defined frame", "64 x 64, 2ms lines", "128 x 128, 2ms lines", "256 x 256, 2ms lines", "512 x 512, 2ms lines", "32 x 32, 1ms lines"] ("Scan format")
            n1807 = call "LoadImagesnewFOCUS.vi"() -> ("Image2Array"=w3141:u8[][], "Image1Array"=w3142:u8[][], "HeaderCluster"=w3199:T21, "Zsin3D"=w3188:sgl[], "ScanLine FreeLine"=w3147:sgl[][], "Image4Array"=w3140:u8[][], "Image3Array"=w3139:u8[][])
            n1808 = Transpose 2D Array(2D array=w3147) -> (transposed array=w3146:sgl[][])
            n1809 = local write "Zsin3D"(w3188) -> ()
            n1810 = local write "ScanLineFreeLine"(w3146) -> ()
            n1811 = local write "frame/line indicator"(w3174) -> ()
            n1812 = local write "Scan format"(w3189) -> ()
            n1813 = Unbundle(w3199) -> ("Program Version"=w3160:u16, "name"=w3198:string, "Time"=w3197:string, "Date"=w3196:string, "start"=w3195:u32, "stop"=w3194:u32, "IntDevUsed"=w3193:bool, "Intensity"=w3192:sgl, "Scan Block Length"=w3191:sgl, "Pixel Clock (Hz)"=w3190:sgl, "X-pixels"=w3158:sgl, "Y-lines"=w3157:sgl, "Number of frames"=w3138:sgl, "Averaging"=w3137:u16, "line scan time (ms)"=w3136:sgl, "Retrace pixels"=w3135:sgl, "z-step (um)"=w3134:sgl, "x-step (um)"=w3133:sgl, "y-step (um)"=w3132:sgl, "x jog"=w3131:sgl, "y jog"=w3130:sgl, "Rotation"=w3129:sgl, "Zoom"=w3128:sgl, "Number of stacks"=w3127:sgl, "Time interval [s]"=w3126:sgl, w3125:T22)  [unwired: 2 out]
            n1814 = Type Cast(type="" ("concatenated string"), x=w3160) -> (*(type *) &x=w3165:string)
            n1815 = local write "Number of Stacks"(w3127) -> ()
            n1816 = local write "Time interval [s]"(w3126) -> ()
            n1817 = String Subset(string=w3165, offset (0)=0, length (rest)=1 ("length (rest)")) -> (substring=w3164:string)
            n1818 = String Subset(string=w3165, offset (0)=1, length (rest)=1 ("length (rest)")) -> (substring=w3163:string)
            n1819 = Concatenate Strings(w3164, "." ("concatenated string"), w3163) -> (w3161:string)
            n1820 = local write "Number of stacks"(w3127) -> ()
            n1821 = local write "Time interval [s]"(w3126) -> ()
            n1822 = local write "Program Version"(w3161) -> ()
            n1823 = local write "Filename"(w3198) -> ()
            n1824 = local write "Number of frames"(w3138) -> ()
            n1825 = local write "Averaging"(w3137) -> ()
            n1826 = local write "Program Version"(w3160) -> ()
            n1827 = local write "Time"(w3197) -> ()
            n1828 = local write "Date"(w3196) -> ()
            n1829 = local write "start"(w3195) -> ()
            n1830 = local write "stop"(w3194) -> ()
            n1831 = local write "IntDevUsed"(w3193) -> ()
            n1832 = local write "Intensity"(w3192) -> ()
            n1833 = local write "Scan Block Length"(w3191) -> ()
            n1834 = local write "Pixel Clock (Hz)"(w3190) -> ()
            n1835 = local write "X-pixels"(w3158) -> ()
            n1836 = local write "Y-lines"(w3157) -> ()
            n1837 = local write "line scan time (ms)"(w3136) -> ()
            n1838 = local write "x-step (um)"(w3133) -> ()
            n1839 = local write "y-step (um)"(w3132) -> ()
            n1840 = local write "x jog"(w3131) -> ()
            n1841 = local write "y jog"(w3130) -> ()
            n1842 = local write "Rotation"(w3129) -> ()
            n1843 = local write "Zoom"(w3128) -> ()
            n1844 = local write "Retrace pixels"(w3135) -> ()
            n1845 = local write "z-step (um)"(w3134) -> ()
            n1846 = local write "Y dim"(w3157) -> ()
            n1847 = local write "X dim"(w3158) -> ()
            n1848 = local write "Averaging"(w3137) -> ()
            n1849 = local write "Number of Frames"(w3138) -> ()
